vi "FPGA UI.vi"() -> ()   [LabVIEW 2025, in "FPGA.lvlib" / "FPGA Instrument.lvclass"]
doc: "Copyright 2017 National Instruments Corporation\n\nLicensed under the Apache License, Version 2.0 (the \"License\"); you may not use this file except in compliance with the License. You may obtain a copy of the License at http://www.apache.org/licenses/LICENSE-2.0\nUnless required by applicable law or agreed to in writing, software distributed under the License is distributed on an \"AS IS\" BASIS, WITHOUT WARRANTIES OR CONDITIONS OF ANY KIND, either express or implied. See the License for the specific language governing permissions and limitations under the License."
uses:
  FPGA Instrument.lvclass
  Users/Public/Documents/Sandia National Labs/TSS Plugin/CEF.lvlibp/Node/NodeRef.ctl
  Users/Public/Documents/Sandia National Labs/TSS Plugin/CEF.lvlibp/Node/CEF_Node.lvclass
  Users/Public/Documents/Sandia National Labs/TSS Plugin/CEF.lvlibp/Node/mainQref.ctl
  Users/Public/Documents/Sandia National Labs/TSS Plugin/CEF.lvlibp/Node/UserEventRef.ctl
  Users/Public/Documents/Sandia National Labs/TSS Plugin/Abstract Engine.lvlibp/Plugin/Abstract/Instrument configuration/Default Instrument.ctl
  FPGA configuration/FPGA Setting.ctl
  FPGA Instrument.lvclass/FPGA Instrument.ctl
  FPGA configuration/FPGA configuration.lvclass/FPGA configuration.ctl
  FPGA configuration/Read FPGA Setting.vi
  FPGA configuration/Write FPGA Setting.vi
  <vilib>/Utility/error.llb/Trim Whitespace One-Sided.vi
  FPGA configuration/FPGA configuration.lvclass
  Users/Public/Documents/Sandia National Labs/TSS Plugin/Abstract Engine.lvlibp/Plugin/Abstract/Instrument configuration/Read Instrument Setting.vi
  Users/Public/Documents/Sandia National Labs/TSS Plugin/Abstract Engine.lvlibp/Plugin/Abstract/Instrument configuration/Write Instrument Setting.vi
  Users/Public/Documents/Sandia National Labs/TSS Plugin/Abstract Engine.lvlibp/Plugin/Abstract/Instrument configuration/Instrument configuration.lvclass
panel:
  in  "FPGA":cluster{"Default":T1, "Setting":T2}={"Default"={"Type"="None", "Address"="None", "SW Alias"="None", "Description"="* Type = Class", "Enabled"=TRUE}, "Setting"={"Numeric"=0.5, "Combo"="", "String"="", "Boolean"=FALSE}} {"Setting"."Numeric" format="%#_f"}
  in  "user event":T3
  in  "main queue":T4
  in  "node ref":T5
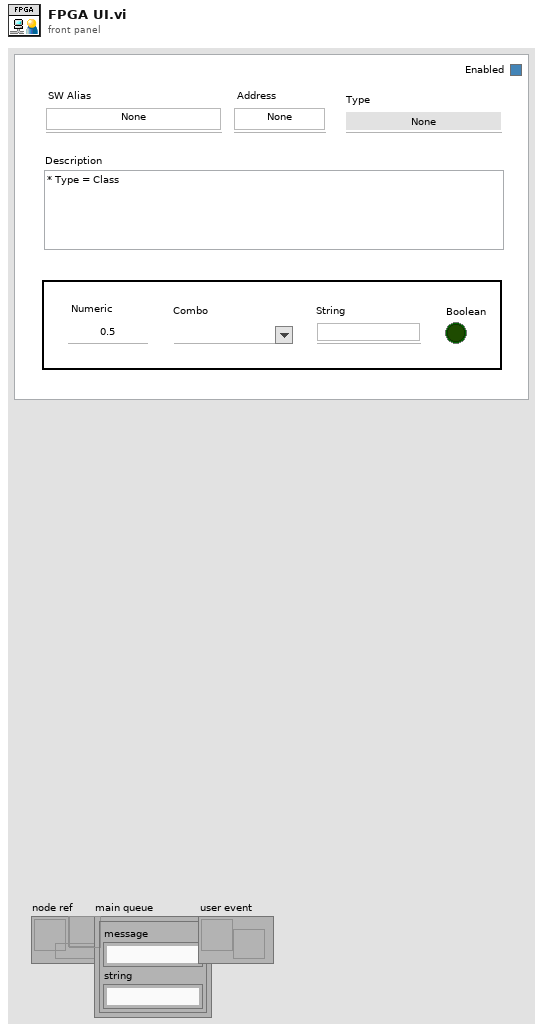
[diagram p1: front panel]
types:
  T1 = typedef "Abstract Engine.lvlibp/Instrument configuration.lvclass/Default Instrument.ctl" = cluster{"Type":string, "Address":string, "SW Alias":string, "Description":string, "Enabled":bool}
  T2 = typedef "FPGA.lvlib/FPGA configuration.lvclass/FPGA Setting.ctl" = cluster{"Numeric":dbl, "Combo":string, "String":string, "Boolean":bool}
  T3 = typedef "CEF.lvlibp/CEF_Node.lvclass/UserEventRef.ctl" = refnum<user-event>
  T4 = typedef "CEF.lvlibp/CEF_Node.lvclass/mainQref.ctl" = refnum<queue>
  T5 = typedef "CEF.lvlibp/CEF_Node.lvclass/NodeRef.ctl" = refnum<data-value>
  T6 = cluster{"Instrument Setting":T1, "FPGA Setting":T2}
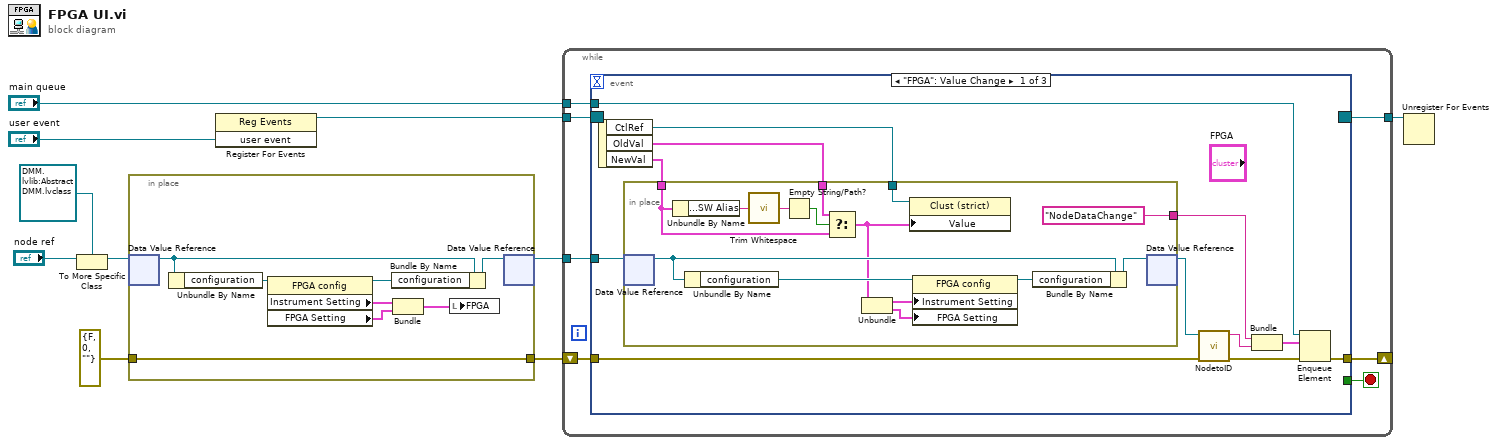
[diagram p0: block diagram]
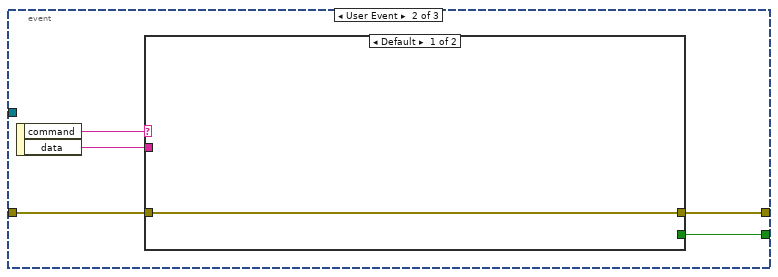
[diagram p2: hidden frame]
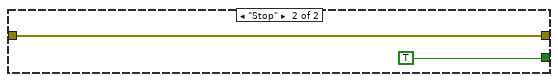
[diagram p3: hidden frame]
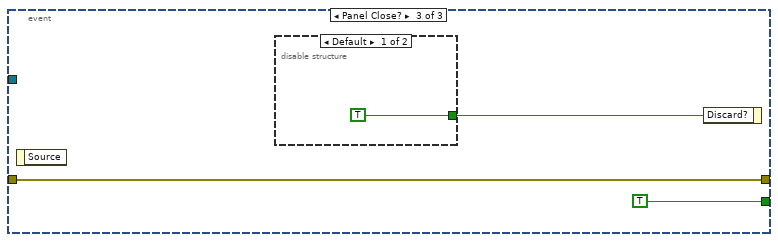
[diagram p4: hidden frame]
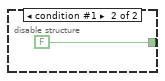
[diagram p5: hidden frame]
diagram:
  n1 = To More Specific Class(target class=refnum<data-value> refnum ("data value reference"), reference="node ref") -> (specific class reference=w7:refnum<data-value>)  [unwired: 1 in, 1 out]
  n2 = in-place {
    in-place-border: errorcluster {"status"=FALSE, "code"=0, "source"=""} ("error out") -> [w11]
    in-place-border: [w11] -> w1
    # "Initialize the front panel controls when loaded"
    n3 = in-place-dvr #1(w7) -> (w17:refnum<class "FPGA Instrument.lvclass">)  [unwired: 1 out]
    n4 = Unbundle By Name(w17) -> ("configuration"=w18:refnum<class "FPGA configuration.lvclass">)
    n5 = property class="FPGA config"(reference=w18) -> (reference out=w16:refnum<class "FPGA configuration.lvclass">, "Instrument Setting"=w14:T1, "FPGA Setting"=w13:T2)  [unwired: 1 in, 1 out]
    n6 = Bundle By Name(cluster=w17, "configuration"=w16) -> (w15:refnum<class "FPGA Instrument.lvclass">)
    n7 = Bundle("Instrument Setting"=w14, "FPGA Setting"=w13) -> (w12:T6)  [unwired: 1 in]
    n8 = local write "FPGA"(w12) -> ()
    n9 = in-place-dvr #1(w15) -> (w6:refnum<data-value>)  [unwired: 1 out]
  }
  n10 = register-events("user event") -> (reference out=w10:refnum<event-registration>)  [unwired: 2 in, 1 out]
  n11 = while {
    tunnel: w6 -> [w25]
    tunnel: w10 -> [w24]
    tunnel: [w23] -> w9
    tunnel: "main queue" -> [w19]
    shift-right: [w20] -> _
    shift-left: w1 -> [w21]
    stop <- w22 stop-if-true
    n12 = event shown="[0] \"FPGA\": Value Change" {
      selector: w24 -> [_ _ _]
      dyn-events: [_ _ _] -> w23
      timeout: _ -> [_ _ _]
      tunnel: w25 -> [w35 _ _]
      tunnel: [_ w56 TRUE] -> w22
      tunnel: [w36 w52 w61] -> w20
      tunnel: w21 -> [w28 w54 w61]
      tunnel: w19 -> [w37 _ _]
      event "FPGA": Value Change {
        n13 = event-data() -> ("CtlRef"=w31:refnum<vi>, "OldVal"=w32:cluster{"Default":T1, "Setting":T2}, "NewVal"=w33:cluster{"Default":T1, "Setting":T2})  [unwired: 1 in]
        n14 = in-place {
          in-place-border: w33 -> [w46]
          in-place-border: w32 -> [w44]
          in-place-border: w31 -> [w43]
          in-place-border: ["NodeDataChange" ("Message Name")] -> w30
          n15 = in-place-dvr #2(w35) -> (w51:refnum<class "FPGA Instrument.lvclass">)  [unwired: 1 out]
          n16 = Unbundle By Name(w46) -> ("Default.SW Alias"=w47:string)
          n17 = Unbundle By Name(w51) -> ("configuration"=w50:refnum<class "FPGA configuration.lvclass">)
          n18 = call <vilib>:"Trim Whitespace.vi"("string"=w47) -> ("trimmed string"=w42:string)  [unwired: 1 in]
          n19 = Empty String/Path?(string/path=w42) -> (empty?=w45:bool)
          n20 = Select(t=w44, s=w45, f=w46) -> (s? t:f=w41:cluster{"Default":T1, "Setting":T2})
          n21 = Unbundle(w41) -> ("Default"=w40:T1, "Setting"=w39:T2)
          n22 = property class="Clust (strict)"(reference=w43, "Value"=w41) -> ()  [unwired: 1 in, 2 out]
          n23 = property class="FPGA config"(reference=w50, "Instrument Setting"=w40, "FPGA Setting"=w39) -> (reference out=w48:refnum<class "FPGA configuration.lvclass">)  [unwired: 1 in, 1 out]
          n24 = Bundle By Name(cluster=w51, "configuration"=w48) -> (w49:refnum<class "FPGA Instrument.lvclass">)
          n25 = in-place-dvr #2(w49) -> (w34:refnum<data-value>)  [unwired: 1 out]
        }
        n26 = call "NodetoID.vi"("error in"=w28, "node ref"=w34) -> ("error out"=w27:errorcluster, "ID"=w29:string)  [unwired: 8 in]
        n27 = Bundle("Message Name"=w30, "ID"=w29) -> (w26:cluster{"Message Name":string, "ID":string})  [unwired: 1 in]
        n28 = Enqueue Element(queue=w37, element=w26, error in (no error)=w27) -> (error out=w36:errorcluster)  [unwired: 1 in, 2 out]
      }
      event User Event {
        n29 = event-data() -> ("command"=w53:string, "data"=w55:string)  [unwired: 1 in]
        n30 = case shown="Default" w53 {
          tunnel: [_ TRUE] -> w56
          tunnel: w55 -> [_ _]
          tunnel: w54 -> [w57 w58]
          tunnel: [w57 w58] -> w52
          frame Default {
          }
          frame "Stop" {
          }
        }
      }
      event Panel Close? {
        n31 = event-data() -> ()  [unwired: 1 in, 1 out]
        n32 = disable-structure shown="Default" {
          disable-tunnel: [TRUE FALSE] -> w60
          frame condition #0 (active) {
          }
          frame condition #1 {
          }
        }
        n33 = event-data("Discard?"=w60) -> ()  [unwired: 1 in, 1 out]
      }
    }
  }
  n34 = Unregister For Events(event registration refnum=w9) -> ()  [unwired: 1 in, 1 out]
